vi "ProcessUDPValues.vi"(8 "error in (no error)":errorcluster, 11 "connection ID":refnum<k16>) -> ()   [LabVIEW 2016]
uses:
  GlobalVars.vi
panel:
  out "ProcessTime":dbl
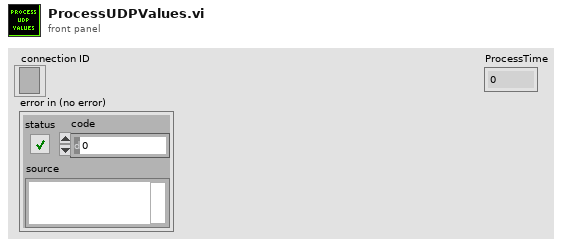
[diagram p1: front panel]
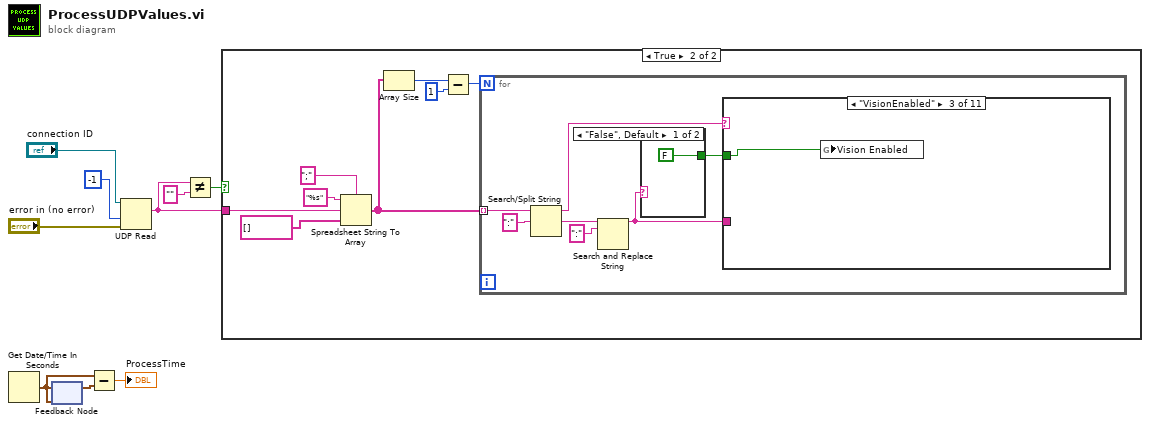
[diagram p0: block diagram]
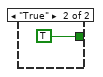
[diagram p3: hidden frame]
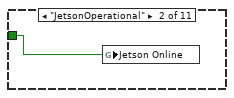
[diagram p5: hidden frame]
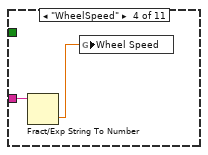
[diagram p6: hidden frame]
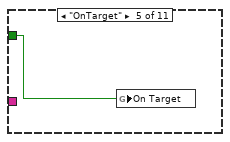
[diagram p7: hidden frame]
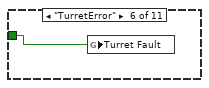
[diagram p8: hidden frame]
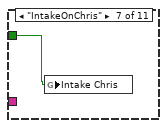
[diagram p9: hidden frame]
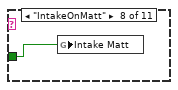
[diagram p10: hidden frame]
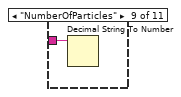
[diagram p11: hidden frame]
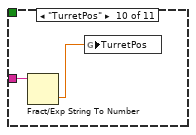
[diagram p12: hidden frame]
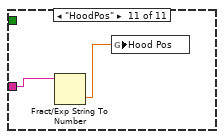
[diagram p13: hidden frame]
diagram:
  n1 = Get Date/Time In Seconds() -> (seconds since 1Jan1904=w7:timestamp)
  n2 = feedback-in #1(w7) -> ()
  n3 = feedback #1(w7) -> (w9:timestamp)
  n4 = Subtract(x=w7, y=w9) -> (x-y=→"ProcessTime":dbl)
  n5 = UDP Read(connection ID="connection ID", timeout ms (25000)=-1, 8:"error in (no error)") -> (data out=w1:string)  [unwired: 1 in, 4 out]
  n6 = Not Equal?(x=w1, y="") -> (x != y?=w2:bool)
  n7 = case shown="True" w2 {
    tunnel: w1 -> [_ w17]
    frame False {
    }
    frame True {
      n8 = Spreadsheet String To Array(delimiter (Tab)=";" ("search string/char (-)"), format string="%s", spreadsheet string=w17, array type (2D Dbl)=string[] []) -> (array=w13:string[])
      n9 = Array Size(array=w13) -> (size(s)=w12:i32)
      n10 = Subtract(x=w12, y=1) -> (x-y=w10:i32)
      n11 = for {
        N: w10 -> [_]
        tunnel: w13 -> [w24] mode=indexing
        n12 = Search/Split String(string=w24, search string/char (-)=":") -> (substring before match=w22:string, match + rest of string=w21:string)  [unwired: 1 in, 1 out]
        n13 = Search and Replace String(input string=w21, search string=":" ("replace string (\"\")")) -> (result string=w19:string)  [unwired: 6 in, 3 out]
        n14 = case shown="\"False\", Default" w19 {
          tunnel: [FALSE TRUE] -> w18
          frame "False", Default {
          }
          frame "True" {
          }
        }
        n15 = case shown="\"VisionEnabled\"" w22 {
          tunnel: w19 -> [_ _ _ w30 _ _ _ _ w35 w37 w38]
          tunnel: w18 -> [_ w27 w28 _ w31 w32 w33 w34 _ _ _]
          frame "False", Default {
          }
          frame "JetsonOperational" {
            n16 = global write "GlobalVars.vi" "Jetson Online"(w27) -> ()
          }
          frame "VisionEnabled" {
            n17 = global write "GlobalVars.vi" "Vision Enabled"(w28) -> ()
          }
          frame "WheelSpeed" {
            n18 = Fract/Exp String To Number(string=w30) -> (number=w29:dbl)  [unwired: 3 in, 1 out]
            n19 = global write "GlobalVars.vi" "Wheel Speed"(w29) -> ()
          }
          frame "OnTarget" {
            n20 = global write "GlobalVars.vi" "On Target"(w31) -> ()
          }
          frame "TurretError" {
            n21 = global write "GlobalVars.vi" "Turret Fault"(w32) -> ()
          }
          frame "IntakeOnChris" {
            n22 = global write "GlobalVars.vi" "Intake Chris"(w33) -> ()
          }
          frame "IntakeOnMatt" {
            n23 = global write "GlobalVars.vi" "Intake Matt"(w34) -> ()
          }
          frame "NumberOfParticles" {
            n24 = Decimal String To Number(string=w35) -> ()  [unwired: 2 in, 2 out]
          }
          frame "TurretPos" {
            n25 = Fract/Exp String To Number(string=w37) -> (number=w36:dbl)  [unwired: 3 in, 1 out]
            n26 = global write "GlobalVars.vi" "TurretPos"(w36) -> ()
          }
          frame "HoodPos" {
            n27 = Fract/Exp String To Number(string=w38) -> (number=w39:dbl)  [unwired: 3 in, 1 out]
            n28 = global write "GlobalVars.vi" "Hood Pos"(w39) -> ()
          }
        }
      }
    }
  }
